vi "Connect.vi"(6 "N attempts":i32=10, 7 "Server parameters":cluster{"IP":string, "Port":u16}={"IP"="28.0.0.0", "Port"=6666}, 8 "Error In":errorcluster, 11 "Local port":u16=3333) -> (0 "Error Out":errorcluster, 3 "connection ID out":refnum<k16>)   [LabVIEW 2016, in "MKR1000.lvlib"]
doc: "This VI (client) trys to start a connection with a Arduino/Genuino MKR1000 (server) through a particular WiFi network N times.\nIP and Port are respectively the IP address and the Port used by MKR1000 to communicate with the VI. Port and local port are set both in MKR firmware and VI. Remember to change both codes to make them work.\n\nNOTE:\nThe MKR1000 VI Library uses UDP. UDP is a connectionless protocol. With the term \"connection\" is intended that MKR1000 gives back an ACKnoledgment packet for each command sent. If no packet is returned (MKR1000 not connected to the net, out of range, etc.), the command is intended LOST and the VIs attempts to send the command again few times before returning Error 5000"
uses:
  MKR1000.lvlib
  Typedef/MKR1000 - Commands.ctl
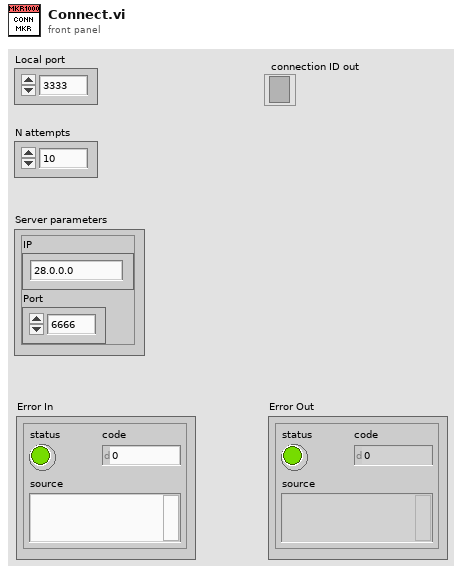
[diagram p1: front panel]
types:
  T1 = typedef "MKR1000.lvlib/MKR1000 - Commands.ctl" = string
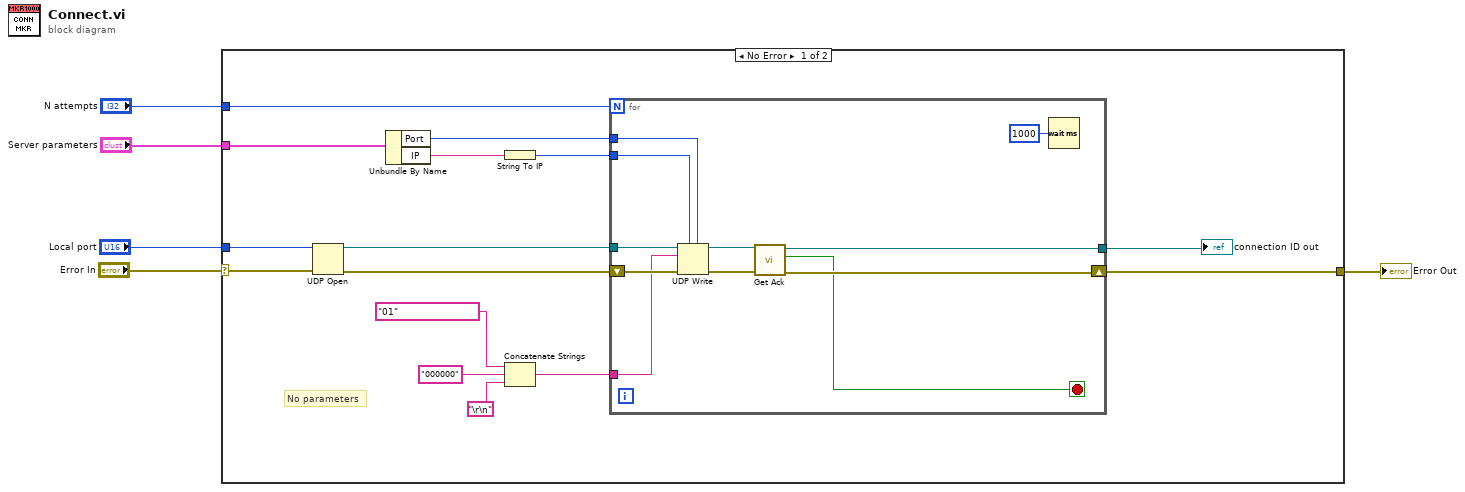
[diagram p0: block diagram]
diagram:
  n1 = case shown="No Error" "Error In" {
    selector: "Error In" -> [w13 w32]
    tunnel: "Server parameters" -> [w19 _]
    tunnel: [w9 w32] -> w3
    tunnel: "Local port" -> [w14 _]
    tunnel: "N attempts" -> [w6 _]
    frame No Error {
      # "No parameters"
      n2 = UDP Open(8:w13, 11:w14) -> (port=w16:refnum<k16>, 0:w15:errorcluster)  [unwired: 3 in, 1 out]
      n3 = Unbundle By Name(w19) -> ("Port"=w17:u16, "IP"=w18:string)
      n4 = String To IP(1:w18) -> (0:w20:u32)
      n5 = Concatenate Strings(T1 "01" ("Command"), "000000" ("string"), "\r\n") -> (w8:string)
      n6 = for {
        N: w6 -> [_]
        tunnel: w20 -> [w31]
        tunnel: w17 -> [w30]
        shift-right: [w23] -> w9
        shift-left: w15 -> [w28]
        tunnel: w16 -> [w29]
        tunnel: w8 -> [w27]
        tunnel: [w22] -> w7
        stop <- w21 stop-if-true
        n7 = UDP Write(address=w31, port or service name=w30, connection ID=w29, data in=w27, 8:w28) -> (error out=w24:errorcluster, 3:w25:refnum<k16>)  [unwired: 1 in]
        n8 = call "Get Ack.vi"("Error In"=w24, "connection ID"=w25) -> ("Error Out"=w23:errorcluster, "Ack status"=w21:bool, "connection ID out"=w22:refnum<k16>)  [unwired: 7 in]
        n9 = Wait (ms)(milliseconds to wait=u32 1000) -> ()  [unwired: 1 out]
      }
      "connection ID out" <- w7
    }
    frame Error {
    }
  }
  "Error Out" <- w3
